vi "Get_Install_Path.vi"(8 "error in (no error)":errorcluster, 10 "IB_Source in":refnum<class "IB_Source.lvclass">, 11 "IB_Tree_Item_Source_Container in":refnum<class "IB_Tree_Item_Source_Container.lvclass">) -> (0 "error out":errorcluster, 2 "eng_installPath":string, 3 "IB_Tree_Item_Source_Container out":refnum<class "IB_Tree_Item_Source_Container.lvclass">)   [LabVIEW 2020, in "IB_Tree_Item_Source_Container.lvclass"]
uses:
  <vilib>/AppBuilder/IB_Classes/Tree_Item_Source_Container/IB_Tree_Item_Source_Container.lvclass
  <vilib>/AppBuilder/IB_Classes/Tree_Item_Source_Container/IB_Tree_Item_Source_Container.lvclass/IB_Tree_Item_Source_Container.ctl
  <vilib>/AppBuilder/IB_Classes/Source/IB_Source.lvclass
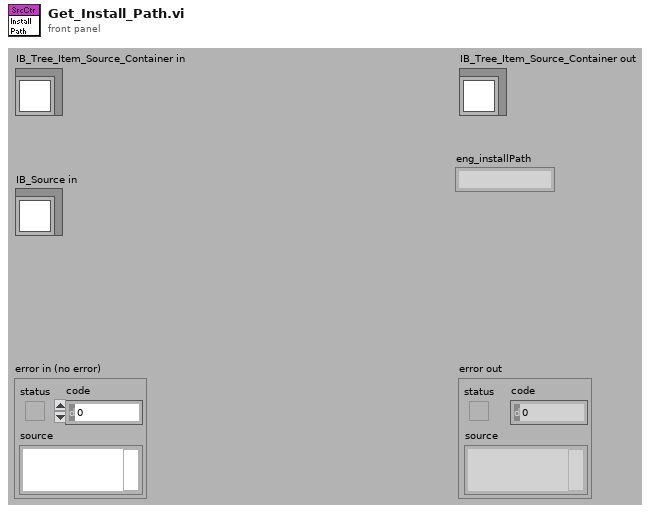
[diagram p1: front panel]
types:
  T1 = typedef "IB_Source.ctl" = cluster{"name":string, "sourceTag":string, "destTag":string, "path":path, "eng_installPath":string, "UI_inBuild?":bool, "str ref?":bool}
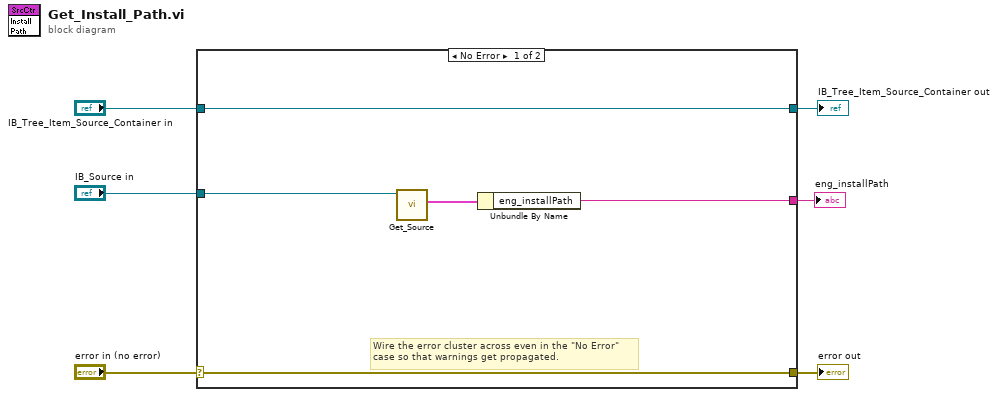
[diagram p0: block diagram]
diagram:
  n1 = case shown="No Error" "error in (no error)" {
    selector: "error in (no error)" -> [w10 w13]
    tunnel: [w10 w13] -> w5
    tunnel: [w11 w12] -> w3
    tunnel: "IB_Tree_Item_Source_Container in" -> [w11 w12]
    tunnel: "IB_Source in" -> [w7 _]
    tunnel: [w8 _] -> w1
    frame No Error {
      # "Wire the error cluster across even in the \"No Error\"\ncase so that warnings get propagated."
      n2 = call <vilib>:"Get_Source.vi"("IB_Source in"=w7) -> ("data"=w9:T1)  [unwired: 1 in, 9 out]
      n3 = Unbundle By Name(w9) -> ("eng_installPath"=w8:string)
    }
    frame Error {
    }
  }
  "error out" <- w5
  "IB_Tree_Item_Source_Container out" <- w3
  "eng_installPath" <- w1
